vi "Display.vi"() -> ()   [LabVIEW 2010, in "Visualizer.lvlib"]
uses:
  Visualizer.lvlib
  Message.ctl
  <vilib>/Waveform/WDTOps.llb/WDT Get Final Time Value DBL.vi
  <vilib>/Waveform/WDTOps.llb/WDT Get Waveform Subset DBL.vi
panel:
  out "Chart":waveform(dbl)[](graph)
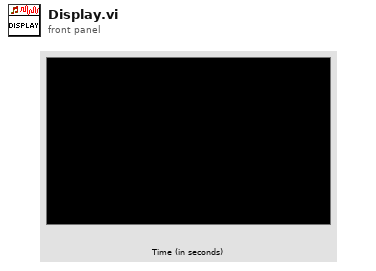
[diagram p1: front panel]
types:
  T1 = typedef "Visualizer.lvlib/Message.ctl" = cluster{"Command":string, "Data":variant}
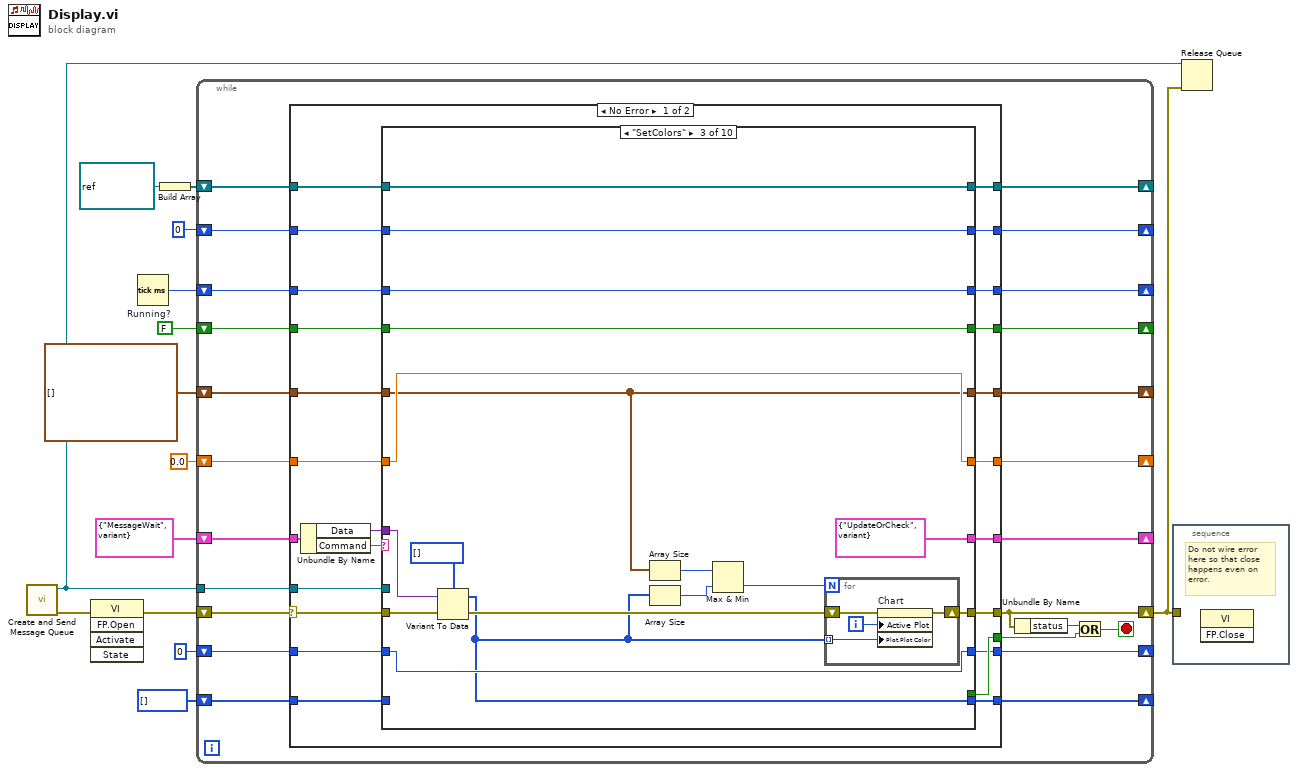
[diagram p0: block diagram]
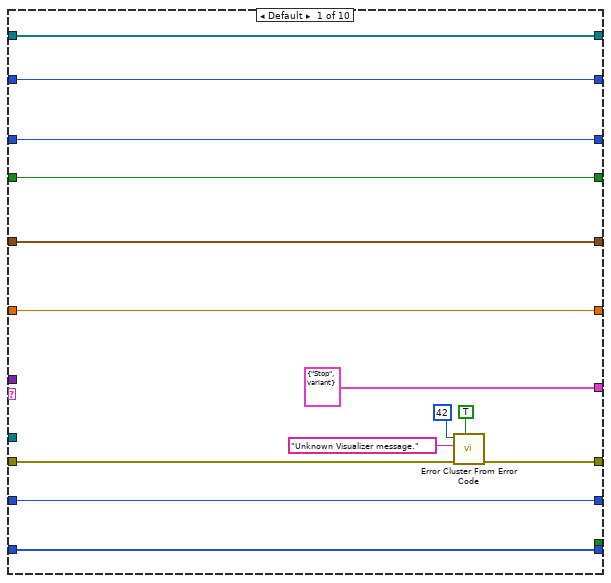
[diagram p2: hidden frame]
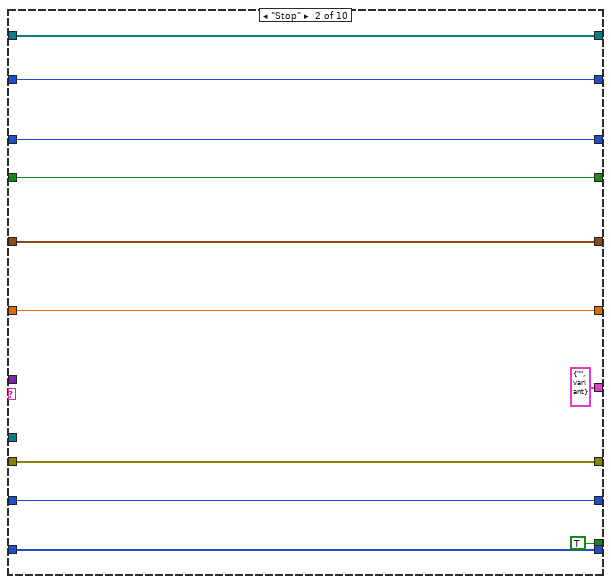
[diagram p3: hidden frame]
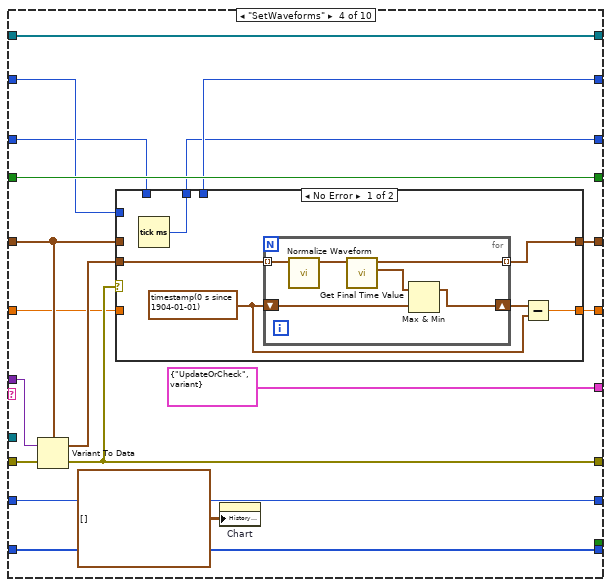
[diagram p4: hidden frame]
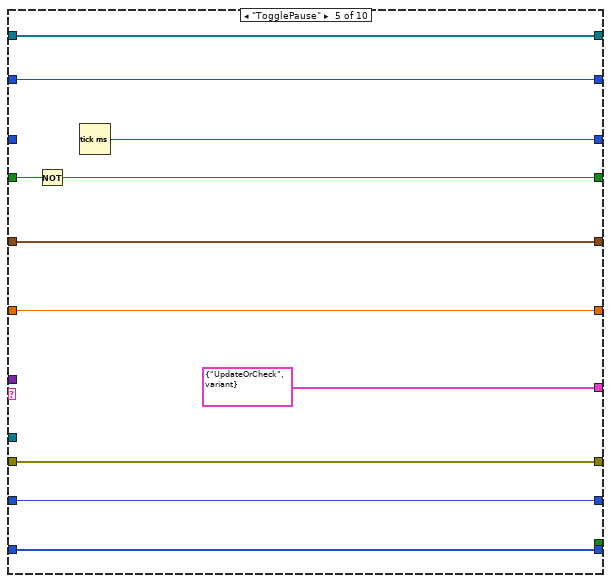
[diagram p6: hidden frame]
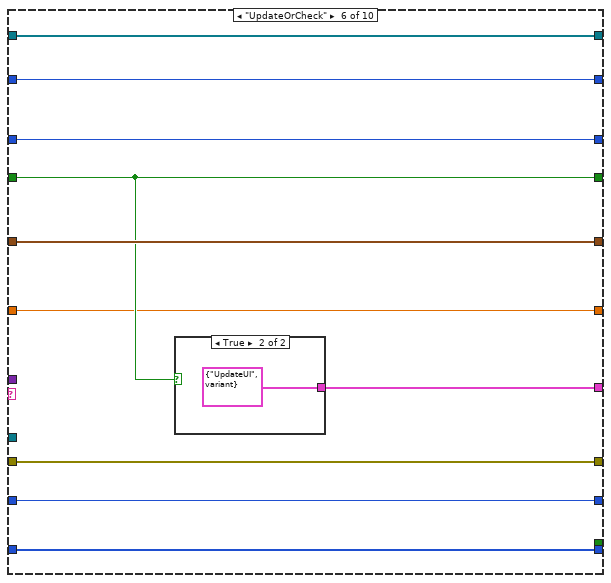
[diagram p7: hidden frame]
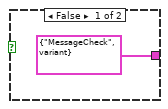
[diagram p8: hidden frame]
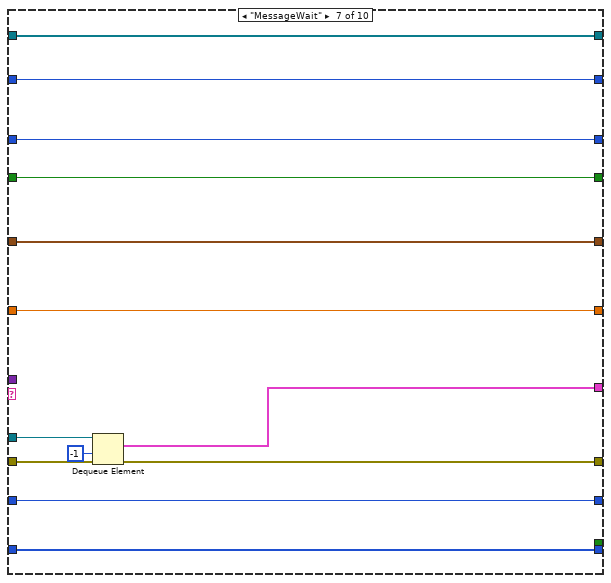
[diagram p9: hidden frame]
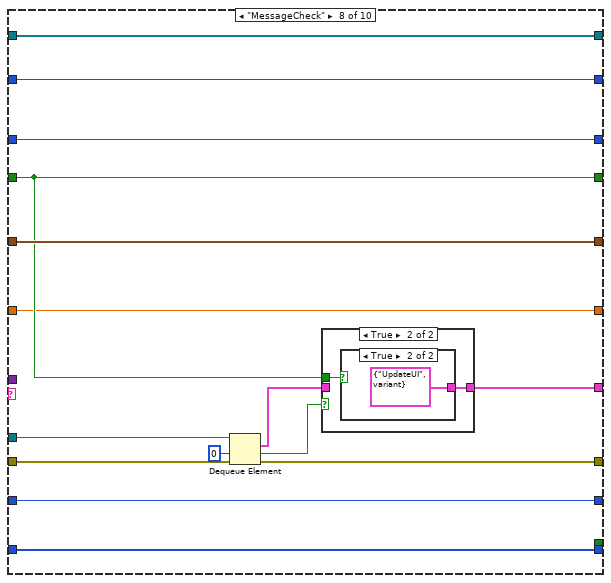
[diagram p10: hidden frame]
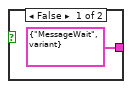
[diagram p12: hidden frame]
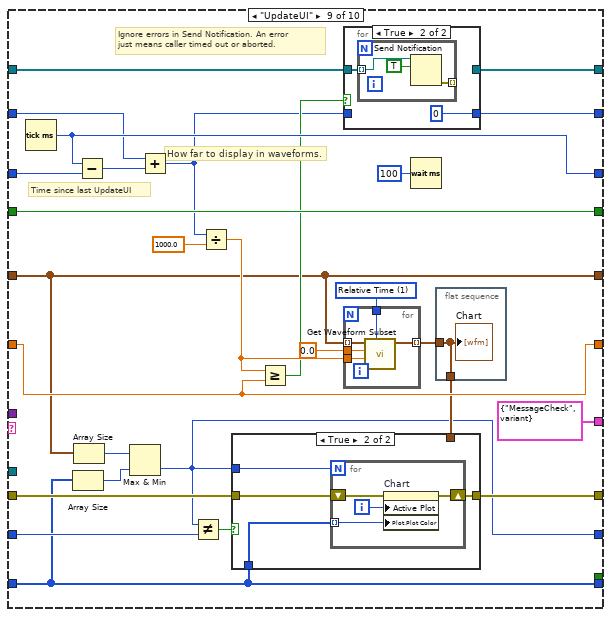
[diagram p13: hidden frame]
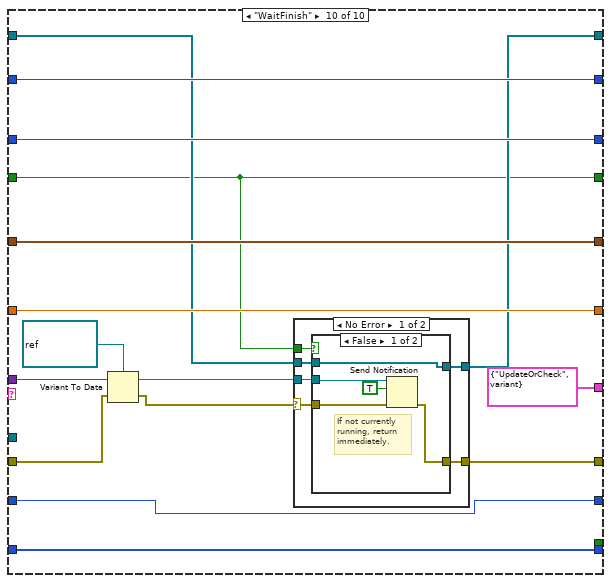
[diagram p16: hidden frame]
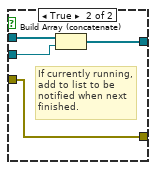
[diagram p17: hidden frame]
diagram:
  w13 = FALSE  # Running?
  n1 = call "Create and Send Message Queue.vi"() -> ("error out"=w11:errorcluster, "queue out"=w9:refnum<queue>)  [unwired: 10 in]
  n2 = invoke class="VI" method="FP.Open"(error in=w11) -> (error out=w10:errorcluster)  [unwired: 4 in, 4 out]
  n3 = Tick Count (ms)() -> (millisecond timer value=w7:u32)
  n4 = Build Array(refnum<notifier> refnum ("notifier out")) -> (w3:refnum<notifier>[])
  n5 = while {
    tunnel: w9 -> [w30]
    shift-right: [w37] -> w14
    shift-left: w10 -> [w29]
    shift-right: [w34] -> _
    shift-left: waveform(dbl)[] [] ("Chart") -> [w33]
    shift-right: [w31] -> _
    shift-left: w13 -> [w32]
    shift-right: [w28] -> _
    shift-left: T1 {"Command"="MessageWait", "Data"=variant} ("Message") -> [w27]
    shift-right: [w24] -> _
    shift-left: w7 -> [w26]
    shift-right: [w23] -> _
    shift-left: u32 0 ("millisecond timer value") -> [w25]
    shift-right: [w22] -> _
    shift-left: 0.0 -> [w21]
    shift-right: [w19] -> _
    shift-left: w3 -> [w20]
    shift-right: [w18] -> _
    shift-left: u32[] [] -> [w17]
    shift-right: [w15] -> _
    shift-left: 0 -> [w16]
    stop <- w35 stop-if-true
    n6 = case shown="No Error" w29 {
      selector: w29 -> [w57 w291]
      tunnel: w27 -> [w62 w288]
      tunnel: [w60 _] -> w38
      tunnel: [w59 w291] -> w37
      tunnel: [w56 w290] -> w34
      tunnel: w33 -> [w55 w290]
      tunnel: w32 -> [w54 w289]
      tunnel: [w53 w289] -> w31
      tunnel: w30 -> [w52 _]
      tunnel: [w51 w288] -> w28
      tunnel: w26 -> [w50 w286]
      tunnel: w25 -> [w49 w287]
      tunnel: [w48 w286] -> w24
      tunnel: [w47 w287] -> w23
      tunnel: [w46 w285] -> w22
      tunnel: w21 -> [w45 w285]
      tunnel: w20 -> [w44 w284]
      tunnel: [w43 w284] -> w19
      tunnel: [w42 w283] -> w18
      tunnel: w17 -> [w41 w283]
      tunnel: w16 -> [w40 w282]
      tunnel: [w39 w282] -> w15
      frame No Error {
        n7 = Unbundle By Name(w62) -> ("Data"=w58:variant, "Command"=w61:string)
        n8 = case shown="\"SetColors\"" w61 {
          tunnel: [w76 w87 w95 w121 w150 w161 w174 w190 w206 w251] -> w59
          tunnel: w57 -> [w75 w87 w103 w125 w150 w161 w175 w191 w207 w258]
          tunnel: [_ TRUE _ _ _ _ _ _ _ _] -> w60
          tunnel: w58 -> [_ _ w104 w126 _ _ _ _ _ w259]
          tunnel: [w74 w85 w94 w124 w153 w163 w178 w193 w208 w264] -> w56
          tunnel: w55 -> [w74 w85 w94 w122 w153 w163 w178 w193 w208 w264]
          tunnel: w54 -> [w73 w84 w101 w120 w152 w160 w177 w185 w226 w252]
          tunnel: [w73 w84 w101 w120 w149 w160 w177 w185 w226 w252] -> w53
          tunnel: w52 -> [_ _ _ _ _ _ w176 w192 _ _]
          tunnel: [T1 {"Command"="Stop", "Data"=variant} ("Message") T1 {"Command"="", "Data"=variant} ("Message") T1 {"Command"="UpdateOrCheck", "Data"=variant} ("Message") T1 {"Command"="UpdateOrCheck", "Data"=variant} ("Message") T1 {"Command"="UpdateOrCheck", "Data"=variant} ("Message") w162 w173 w186 T1 {"Command"="MessageCheck", "Data"=variant} ("Message") T1 {"Command"="UpdateOrCheck", "Data"=variant} ("Message")] -> w51
          tunnel: w50 -> [w67 w81 w98 w113 _ w158 w170 w183 w223 w263]
          tunnel: w49 -> [w68 w82 w99 w115 w147 w159 w171 w184 w220 w262]
          tunnel: [w67 w81 w98 w112 w148 w158 w170 w183 w222 w263] -> w48
          tunnel: [w68 w82 w99 w114 w147 w159 w171 w184 w212 w262] -> w47
          tunnel: [w66 w80 w97 w118 w146 w157 w169 w182 w214 w261] -> w46
          tunnel: w45 -> [w66 w80 w97 w117 w146 w157 w169 w182 w214 w261]
          tunnel: w44 -> [w65 w79 w96 w111 w145 w156 w168 w181 w210 w256]
          tunnel: [w65 w79 w96 w111 w145 w156 w168 w181 w209 w254] -> w43
          tunnel: [w64 w78 w91 w110 w144 w155 w167 w180 w202 w250] -> w42
          tunnel: w41 -> [w64 w78 _ w110 w144 w155 w167 w180 w202 w250]
          tunnel: w40 -> [w63 w77 w92 w109 w143 w154 w166 w179 w205 w249]
          tunnel: [w63 w77 w92 w109 w143 w154 w166 w179 w199 w249] -> w39
          frame Default {
            n9 = call <vilib>:"Error Cluster From Error Code.vi"("show call chain? (False)"=TRUE, "error in (no error)"=w75, "error message (\"\")"="Unknown Visualizer message." ("error message (\"\")"), "error code (0)"=42) -> ("error out"=w76:errorcluster)  [unwired: 5 in]
          }
          frame "Stop" {
          }
          frame "SetColors" {
            n10 = Variant To Data(error in=w103, Variant=w104, type=u32[] []) -> (error out=w93:errorcluster, data=w91:u32[])
            n11 = Array Size(array=w94) -> (size(s)=w90:i32)
            n12 = Array Size(array=w91) -> (size(s)=w89:i32)
            n13 = Max & Min(x=w90, y=w89) -> (min(x,y)=w88:i32)  [unwired: 1 out]
            n14 = for {
              N: w88 -> [_]
              shift-right: [w106] -> w95
              shift-left: w93 -> [w107]
              tunnel: w91 -> [w105] mode=indexing
              i -> [w108]
              n15 = property on="Chart" class="WFChart (strict)"(error in=w107, "Active Plot"=w108, "Plot.Plot Color"=w105) -> (error out=w106:errorcluster)  [unwired: 1 in, 1 out]
            }
          }
          frame "SetWaveforms" {
            n16 = Variant To Data(error in=w125, Variant=w126, type=w122) -> (error out=w121:errorcluster, data=w123:waveform(dbl)[])
            n17 = case shown="No Error" w121 {
              tunnel: [w131 w142] -> w124
              tunnel: w123 -> [w132 _]
              tunnel: w122 -> [_ w142]
              tunnel: [w129 w141] -> w118
              tunnel: w117 -> [_ w141]
              tunnel: w115 -> [_ w140]
              tunnel: [_ w140] -> w114
              tunnel: w113 -> [_ w139]
              tunnel: [w127 w139] -> w112
              frame No Error {
                w128 = timestamp(0 s since 1904-01-01) ("tf")
                n18 = Tick Count (ms)() -> (millisecond timer value=w127:u32)
                n19 = for {
                  tunnel: w132 -> [w138] mode=indexing
                  tunnel: [w137] -> w131 mode=indexing
                  shift-right: [w133] -> w130
                  shift-left: w128 -> [w134]
                  n20 = call <vilib>:"Normalize Waveform.vi"("waveform in"=w138) -> ("normalized waveform"=w136:waveform(dbl))  [unwired: 7 in, 3 out]
                  n21 = call-poly <vilib>:"Get Final Time Value.vi"("waveform in"=w136) -> ("tf"=w135:timestamp, "waveform out"=w137:waveform(dbl))  [unwired: 8 in, 1 out]
                  n22 = Max & Min(x=w135, y=w134) -> (max(x,y)=w133:timestamp)  [unwired: 1 out]
                }
                n23 = Subtract(x=w130, y=w128) -> (x-y=w129:dbl)
              }
              frame Error {
                # "On error, keep\nprevious value."
              }
            }
            n24 = property on="Chart" class="WFChart (strict)"("History Data"=waveform(dbl)[][] []) -> ()  [unwired: 2 in, 2 out]
          }
          frame "TogglePause" {
            n25 = Not(x=w152) -> (.not. x?=w149:bool)
            n26 = Tick Count (ms)() -> (millisecond timer value=w148:u32)
          }
          frame "UpdateOrCheck" {
            n27 = case shown="True" w160 {
              tunnel: [T1 {"Command"="MessageCheck", "Data"=variant} ("Message") T1 {"Command"="UpdateUI", "Data"=variant} ("Message")] -> w162
              frame False {
              }
              frame True {
              }
            }
          }
          frame "MessageWait" {
            n28 = Dequeue Element(queue=w176, timeout in ms (-1)=-1, error in (no error)=w175) -> (element=w173:T1, error out=w174:errorcluster)  [unwired: 2 out]
          }
          frame "MessageCheck" {
            n29 = Dequeue Element(queue=w192, timeout in ms (-1)=0, error in (no error)=w191) -> (element=w187:T1, timed out?=w188:bool, error out=w190:errorcluster)  [unwired: 1 out]
            n30 = case shown="True" w188 {
              tunnel: w187 -> [w194 _]
              tunnel: [w194 w195] -> w186
              tunnel: w185 -> [_ w196]
              frame False {
              }
              frame True {
                n31 = case shown="True" w196 {
                  tunnel: [T1 {"Command"="MessageWait", "Data"=variant} ("Message") T1 {"Command"="UpdateUI", "Data"=variant} ("Message")] -> w195
                  frame False {
                  }
                  frame True {
                  }
                }
              }
            }
          }
          frame "UpdateUI" {
            w216 = u16 1 items=["Samples", "Relative Time"] ("start/duration format")
            # "Ignore errors in Send Notification. An error\njust means caller timed out or aborted."
            # "How far to display in waveforms."
            # "Time since last UpdateUI"
            n32 = Tick Count (ms)() -> (millisecond timer value=w222:u32)
            n33 = Array Size(array=w202) -> (size(s)=w200:i32)
            n34 = Array Size(array=w208) -> (size(s)=w201:i32)
            n35 = Subtract(x=w222, y=w223) -> (x-y=w221:u32)
            n36 = Max & Min(x=w201, y=w200) -> (min(x,y)=w199:i32)  [unwired: 1 out]
            n37 = Add(x=w220, y=w221) -> (x+y=w211:u32)
            n38 = Not Equal?(x=w199, y=w205) -> (x != y?=w204:bool)
            n39 = Divide(x=w211, y=1000.0 ("start samples/time")) -> (x/y=w215:dbl)
            n40 = case shown="True" w204 {
              tunnel: w202 -> [_ w229]
              tunnel: w207 -> [w227 w231]
              tunnel: [w227 w230] -> w206
              tunnel: w199 -> [_ w228]
              tunnel: w203 -> [_ _]
              frame False {
              }
              frame True {
                n41 = for {
                  N: w228 -> [_]
                  shift-right: [w233] -> w230
                  shift-left: w231 -> [w234]
                  tunnel: w229 -> [w232] mode=indexing
                  i -> [w235]
                  n42 = property on="Chart" class="WFChart (strict)"(error in=w234, "Active Plot"=w235, "Plot.Plot Color"=w232) -> (error out=w233:errorcluster)  [unwired: 1 in, 1 out]
                }
              }
            }
            n43 = Greater Or Equal?(x=w215, y=w214) -> (x >= y?=w213:bool)
            n44 = case shown="True" w213 {
              tunnel: [w238 u32 0] -> w212
              tunnel: w211 -> [w238 _]
              tunnel: w210 -> [w237 w239]
              tunnel: [w237 _] -> w209
              frame False {
              }
              frame True {
                n45 = for {
                  tunnel: w239 -> [w243] mode=indexing
                  tunnel: [w241] -> _ mode=indexing
                  n46 = Send Notification(notification=TRUE, notifier=w243) -> (error out=w241:errorcluster)  [unwired: 1 in, 1 out]
                }
              }
            }
            n47 = for {
              tunnel: 0.0 ("start samples/time") -> [w248]
              tunnel: w215 -> [w247]
              tunnel: w208 -> [w246] mode=indexing
              tunnel: [w245] -> w218 mode=indexing
              tunnel: w216 -> [w244]
              n48 = call-poly <vilib>:"Get Waveform Subset.vi"("start/duration format"=w244, "duration"=w247, "start samples/time"=w248, "waveform in"=w246) -> ("waveform out"=w245:waveform(dbl))  [unwired: 2 in, 3 out]
            }
            n49 = Wait (ms)(milliseconds to wait=u32 100) -> ()  [unwired: 1 out]
            n50 = flat-sequence {
              tunnel: w218 -> [w236]
              tunnel: [w236] -> w203
              frame #0 {
                "Chart" <- w236
              }
            }
          }
          frame "WaitFinish" {
            n51 = Variant To Data(error in=w258, Variant=w259, type=refnum<notifier> refnum ("notifier out")) -> (error out=w253:errorcluster, data=w255:refnum<notifier>)
            n52 = case shown="No Error" w253 {
              selector: w253 -> [w266 w280]
              tunnel: w256 -> [w270 w281]
              tunnel: w255 -> [w269 _]
              tunnel: [w268 w281] -> w254
              tunnel: w252 -> [w267 _]
              tunnel: [w265 w280] -> w251
              frame No Error {
                n53 = case shown="False" w267 {
                  tunnel: w270 -> [w275 w279]
                  tunnel: w269 -> [w274 w278]
                  tunnel: [w275 w277] -> w268
                  tunnel: w266 -> [w272 w276]
                  tunnel: [w271 w276] -> w265
                  frame False {
                    # "If not currently\nrunning, return\nimmediately."
                    n54 = Send Notification(notification=TRUE, notifier=w274, error in (no error)=w272) -> (error out=w271:errorcluster)  [unwired: 1 out]
                  }
                  frame True {
                    # "If currently running,\nadd to list to be\nnotified when next\nfinished."
                    n55 = Build Array (concatenate)(w279, w278) -> (w277:refnum<notifier>[])
                  }
                }
              }
              frame Error {
              }
            }
          }
        }
      }
      frame Error {
      }
    }
    n56 = Unbundle By Name(w37) -> ("status"=w36:bool)
    n57 = Or(x=w36, y=w38) -> (x .or. y?=w35:bool)
  }
  n58 = stacked-sequence {
    tunnel: w14 -> [_]
    frame #0 {
      # "Do not wire error\nhere so that close\nhappens even on\nerror."
      n59 = invoke class="VI" method="FP.Close"() -> ()  [unwired: 3 in, 3 out]
    }
  }
  n60 = Release Queue(queue=w9, error in (no error)=w14) -> ()  [unwired: 1 in, 3 out]
